vi "Test Write Data.vi"() -> ()   [LabVIEW 2020, in "Terminal.lvlib" / "Terminal.lvclass"]
uses:
  Terminal.lvclass
  Terminal.lvclass/Terminal.ctl
panel:
  out "Parse Time":dbl format="%#_6f"
  out "Draw Time":dbl format="%#_6f"
  out "2D Picture":picture
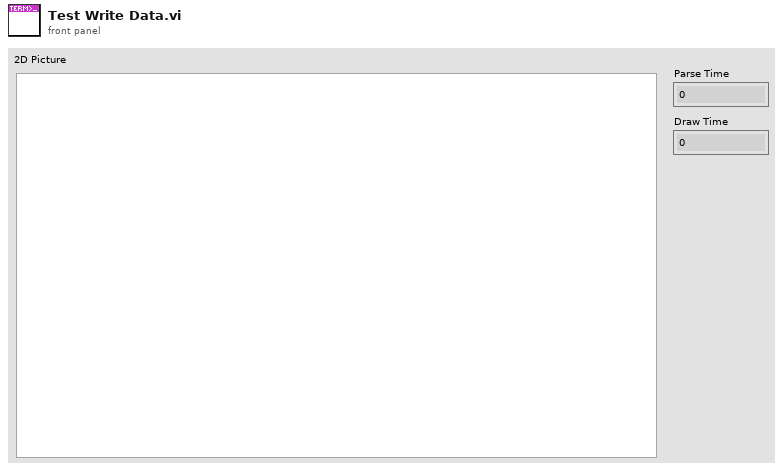
[diagram p1: front panel]
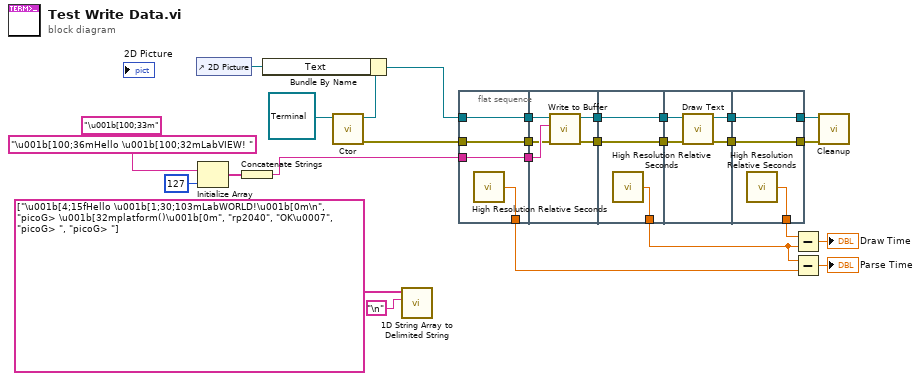
[diagram p0: block diagram]
diagram:
  (unwired) "\u001b[100;33m"
  n1 = control-ref of="2D Picture"() -> (w26:refnum<vi>)
  n2 = Initialize Array("\u001b[100;36mHello \u001b[100;32mLabVIEW! ", 127 ("dimension size")) -> (w2:string[])
  n3 = Concatenate Strings(w2) -> (w1:string)
  n4 = call-dynamic "Ctor.vi"("Terminal in"=refnum<class "Terminal.lvclass"> refnum) -> ("error out"=w25:errorcluster, "Terminal out"=w24:refnum<class "Terminal.lvclass">)  [unwired: 9 in]
  n5 = Bundle By Name(cluster=w24, "Text"=w26) -> (w23:refnum<class "Terminal.lvclass">)
  n6 = call <vilib>:"1D String Array to Delimited String.vi"("delimiter"="\n", "string array"=string[] ["\u001b[4;15fHello \u001b[1;30;103mLabWORLD!\u001b[0m\n", "picoG> \u001b[32mplatform()\u001b[0m", "rp2040", "OK\u0007", "picoG> ", "picoG> "]) -> ()  [unwired: 9 in, 1 out]
  n7 = flat-sequence {
    tunnel: w23 -> [w29]
    tunnel: w25 -> [w30]
    tunnel: w1 -> [w31]
    tunnel: [w31] -> w22
    tunnel: [w30] -> w21
    tunnel: [w29] -> w20
    tunnel: [w28] -> w9
    tunnel: w22 -> [w36]
    tunnel: w21 -> [w35]
    tunnel: w20 -> [w34]
    tunnel: [w33] -> w16
    tunnel: [w32] -> w14
    tunnel: [w39] -> w17
    tunnel: w16 -> [w39]
    tunnel: [w38] -> w15
    tunnel: w14 -> [w38]
    tunnel: [w37] -> w10
    tunnel: w17 -> [w41]
    tunnel: w15 -> [w40]
    tunnel: [w43] -> w13
    tunnel: [w42] -> w12
    tunnel: [w45] -> w18
    tunnel: [w46] -> w19
    tunnel: w13 -> [w46]
    tunnel: w12 -> [w45]
    tunnel: [w44] -> w11
    frame #0 {
      n8 = call <vilib>:"High Resolution Relative Seconds.vi"() -> ("relative seconds"=w28:dbl)
    }
    frame #1 {
      n9 = call "Write to Buffer.vi"("error in (no error)"=w35, "Data"=w36, "Terminal in"=w34) -> ("error out"=w32:errorcluster, "Terminal out"=w33:refnum<class "Terminal.lvclass">)  [unwired: 7 in]
    }
    frame #2 {
      n10 = call <vilib>:"High Resolution Relative Seconds.vi"() -> ("relative seconds"=w37:dbl)
    }
    frame #3 {
      n11 = call "Draw Text.vi"("error in (no error)"=w40, "Terminal in"=w41) -> ("error out"=w43:errorcluster, "Terminal out"=w42:refnum<class "Terminal.lvclass">)  [unwired: 8 in]
    }
    frame #4 {
      n12 = call <vilib>:"High Resolution Relative Seconds.vi"() -> ("relative seconds"=w44:dbl)
    }
  }
  n13 = Subtract(x=w11, y=w10) -> (x-y=→"Draw Time":dbl)
  n14 = Subtract(x=w10, y=w9) -> (x-y=→"Parse Time":dbl)
  n15 = call-dynamic "Cleanup.vi"("error in (no error)"=w19, "Terminal in"=w18) -> ()  [unwired: 9 in, 1 out]
